vi "Ziffernanzeige.vi"(9 "Param Ziffernanzeige":T1={"Wert-String"="123,4567", "Rechteck"={"left"=10, "top"=10, "right"=90, "bottom"=30}, "Schriftgröße"=18, "Textfarbe"=16776769, "Hintergrund"=16730368, "Rahmenfarbe"=16730368}, 11 "Bild":picture caption="Grafik") -> (3 "Bild neu":picture)   [LabVIEW 2020, in "Anlagenuebersicht.lvlib" / "VisBx Anzeige.lvlib"]
uses:
  VisBx Anzeige.lvlib
  VisParameter/Param Ziffernanzeige.ctl
  VisParameter/VisParam-Typdef.lvlib
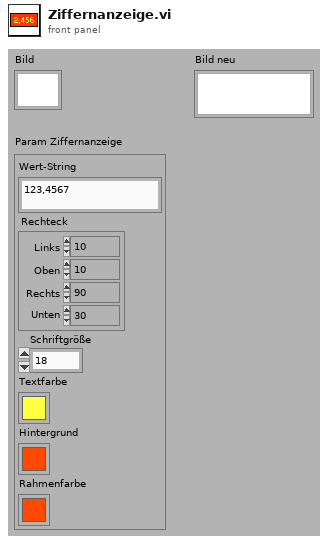
[diagram p1: front panel]
types:
  T1 = typedef "VisParam-Typdef.lvlib/Param Ziffernanzeige.ctl" = cluster{"Wert-String":string, "Rechteck":cluster{"left":i16, "top":i16, "right":i16, "bottom":i16}, "Schriftgröße":i16, "Textfarbe":u32, "Hintergrund":u32, "Rahmenfarbe":u32}
  T2 = cluster{"horizontal":enum16{"left", "center", "right"}, "vertical":enum16{"top", "center", "bottom"}}
  T3 = cluster{"left":i16, "top":i16, "right":i16, "bottom":i16}
  T4 = cluster{"Font Name:":string, "Size":i16, "Strikeout?":bool, "Italic?":bool, "Underline?":bool, "Outline?":bool, "Shadow?":bool, "Bold?":bool}
  T5 = enum16{"User-specified Font", "Application Font", "System Font", "Dialog Font"}
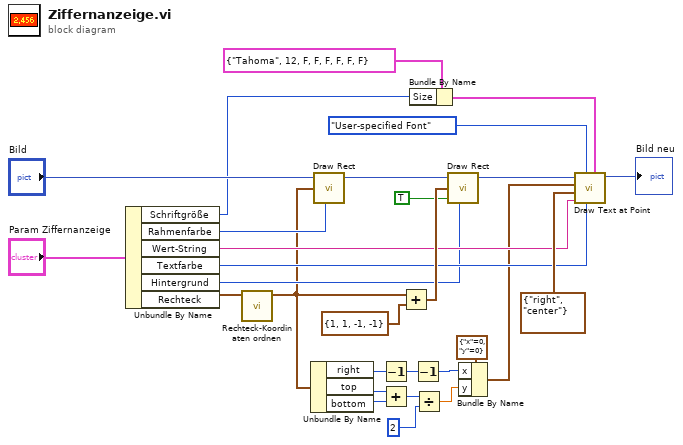
[diagram p0: block diagram]
diagram:
  n1 = Unbundle By Name("Param Ziffernanzeige") -> ("Schriftgröße"=w24:i16, "Rahmenfarbe"=w23:u32, "Wert-String"=w19:string, "Textfarbe"=w18:u32, "Hintergrund"=w13:u32, "Rechteck"=w1:T3)
  n2 = call "Rechteck-Koordinaten ordnen.vi"("Rechteck-Koordinaten"=w1) -> ("Koordinaten geordnet"=w2:T3)  [unwired: 6 in]
  n3 = Unbundle By Name(w2) -> ("right"=w14:i16, "top"=w6:i16, "bottom"=w7:i16)
  n4 = call <vilib>:"Draw Rect.vi"("picture"="Bild", "rect"=w2, "color(black)"=w23) -> ("new picture"=w17:picture)  [unwired: 2 in, 4 out]
  n5 = Decrement(x=w14) -> (x-1=w9:i16)
  n6 = Add(x=w6, y=w7) -> (x+y=w5:i16)
  n7 = Add(x=w2, y=T3 {"left"=1, "top"=1, "right"=-1, "bottom"=-1} ("Rechteck")) -> (x+y=w28:T3)
  n8 = Bundle By Name(cluster=T4 {"Font Name:"="Tahoma", "Size"=12, "Strikeout?"=FALSE, "Italic?"=FALSE, "Underline?"=FALSE, "Outline?"=FALSE, "Shadow?"=FALSE, "Bold?"=FALSE} ("[user-specified font]"), "Size"=w24) -> (w22:T4)
  n9 = Decrement(x=w9) -> (x-1=w8:i16)
  n10 = Divide(x=w5, y=i16 2) -> (x/y=w3:dbl)
  n11 = call <vilib>:"Draw Rect.vi"("picture"=w17, "rect"=w28, "fill?(F)"=TRUE, "color(black)"=w13) -> ("new picture"=w11:picture)  [unwired: 5 in]
  n12 = Bundle By Name(cluster=cluster{"x":i16, "y":i16} {"x"=0, "y"=0} ("origin"), "x"=w8, "y"=w3) -> (w15:cluster{"x":i16, "y":i16})
  n13 = call <vilib>:"Draw Text at Point.vi"("[user-specified font]"=w22, "text color(black)"=w18, "desired font(Application)"=T5."User-specified Font", "text"=w19, "alignment(left, top)"=T2 {"horizontal"=enum."right", "vertical"=enum."center"}, "origin"=w15, "picture"=w11) -> ("new picture"=→"Bild neu":picture)  [unwired: 3 in, 1 out]
